vi "Auto Undeploy Service.vi"() -> ()   [LabVIEW 2016]
uses:
  <vilib>/NI Veristand/Execution/Workspace/NI_VS Workspace ExecutionAPI.lvlib
panel:
  out "Workspace Event":string
  in  "NIVS.Workspace Event":refnum<event-registration>
  in  "NIVS.Project File Path":path
  in  "NIVS.Gateway IP Address":string
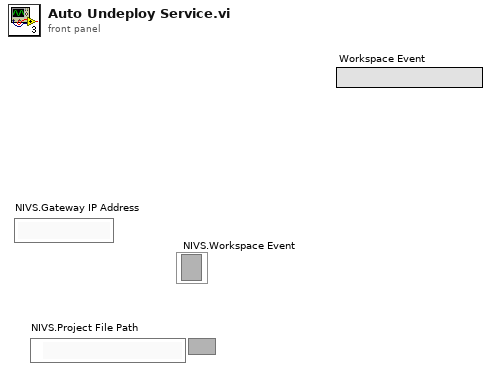
[diagram p1: front panel]
types:
  T1 = typedef "NI_VS Workspace ExecutionAPI.lvlib/WorkspaceAPI.ctl" = refnum<k24>
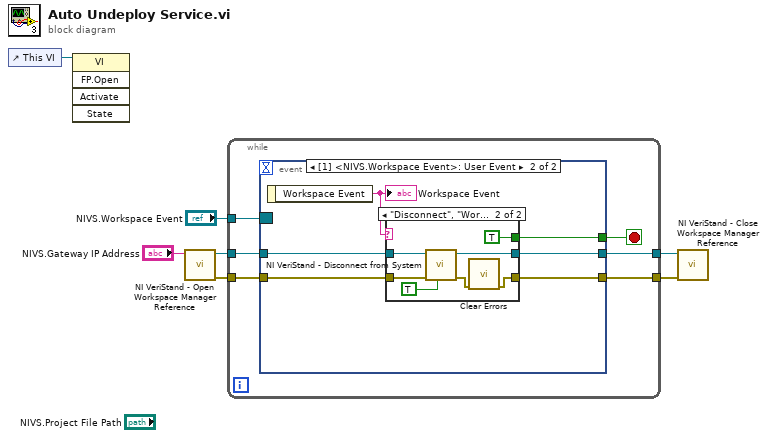
[diagram p0: block diagram]
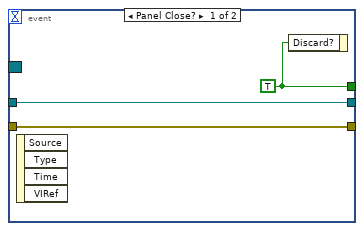
[diagram p2: hidden frame]
diagram:
  n1 = control-ref of="This VI"() -> (w5:refnum<vi>)
  n2 = invoke class="VI" method="FP.Open"(reference=w5) -> ()  [unwired: 4 in, 5 out]
  n3 = call <vilib>:"NI VeriStand - Open Workspace Manager Reference.vi"("Gateway IP Address (\"\": localhost)"="NIVS.Gateway IP Address") -> ("error out"=w3:errorcluster, "WorkspaceManager"=w4:T1)  [unwired: 9 in]
  n4 = while {
    tunnel: "NIVS.Workspace Event" -> [w12]
    tunnel: w4 -> [w11]
    tunnel: w3 -> [w10]
    tunnel: [w9] -> w2
    tunnel: [w8] -> w1
    stop <- w13 stop-if-true
    n5 = event shown="[1] <NIVS.Workspace Event>: User Event" {
      selector: w12 -> [_ _]
      dyn-events: _ -> [_ _]
      timeout: _ -> [_ _]
      tunnel: [w16 w21] -> w13
      tunnel: w11 -> [w15 w20]
      tunnel: w10 -> [w14 w19]
      tunnel: [w15 w18] -> w9
      tunnel: [w14 w17] -> w8
      event Panel Close? {
        w16 = TRUE ("Discard?")
        n6 = event-data() -> ()  [unwired: 1 in, 4 out]
        n7 = event-data("Discard?"=w16) -> ()  [unwired: 1 in, 1 out]
      }
      event User Event {
        n8 = event-data() -> ("Workspace Event"=w22:string)  [unwired: 1 in]
        "Workspace Event" <- w22
        n9 = case shown="\"Disconnect\", \"Workspace.Close\"" w22 {
          tunnel: [_ TRUE] -> w21
          tunnel: w20 -> [w24 w30]
          tunnel: w19 -> [w23 w29]
          tunnel: [w24 w28] -> w18
          tunnel: [w23 w26] -> w17
          frame Default {
          }
          frame "Disconnect", "Workspace.Close" {
            n10 = call <vilib>:"NI VeriStand - Disconnect from System.vi"("Undeploy System Definition (F)"=TRUE, "error in (no error)"=w29, "WorkspaceManager in"=w30) -> ("error out"=w27:errorcluster, "WorkspaceManager out"=w28:T1)  [unwired: 7 in]
            n11 = call <vilib>:"Clear Errors.vi"("error in (no error)"=w27) -> ("error out"=w26:errorcluster)  [unwired: 5 in, 1 out]
          }
        }
      }
    }
  }
  n12 = call <vilib>:"NI VeriStand - Close Workspace Manager Reference.vi"("error in (no error)"=w1, "WorkspaceManager"=w2) -> ()  [unwired: 9 in, 1 out]
